vi "Import-Export_Service.vi"() -> ()   [LabVIEW 2014]
uses:
  _subVIs/_typedefs/impExp_Data.ctl
  <vilib>/NI Veristand/Templates/Workspace Tool Support/Workspace Tool Message Bus.ctl
  <vilib>/NI Veristand/Templates/Workspace Tool Support/Workspace Tool Message (String).ctl
  <vilib>/NI Veristand/Templates/Workspace Tool Support/Workspace Tool Response (String).ctl
  <vilib>/NI Veristand/Templates/Workspace Tool Support/Workspace Tool Message (Byte Array).ctl
  <vilib>/NI Veristand/Templates/Workspace Tool Support/Workspace Tool Response (Byte Array).ctl
  _subVIs/_typedefs/impExp_Service-StateData.ctl
  <vilib>/NI Veristand/Execution/Project/Project Ref.ctl
  _subVIs/Progress Bar/_typedefs/PB_Manager Actions.ctl
  <vilib>/NI/AMC/Create Single Message.vi
  <vilib>/NI/AMC/Update Message Routing Info.vi
  <vilib>/NI/AMC/Read Termination Message.vi
  <vilib>/NI/AMC/Send Message.vi
  <vilib>/NI/AMC/Globals.vi
  <vilib>/NI/AMC/AMC.lvlib
  NationalInstruments.VeriStand.ClientAPI
  <vilib>/NI Veristand/Execution/Project/NI_VS Project ExecutionAPI.lvlib
  <vilib>/NI VeriStand/Execution/Workspace/NI_VS Workspace ExecutionAPI.lvlib
  <vilib>/NI Veristand/Execution/Project/NI VeriStand - Send Workspace Tool Message (String).vi
  _subVIs/Progress Bar/Progress Bar.lvlib
  <vilib>/NI VeriStand/Templates/Workspace Tool Support/NI VeriStand - Workspace Tool Support.lvlib
panel:
  out "NIVS.Project File Path":path
  out "Workspace Events":i32
  in  "New Project/Screen Prefix":string="Proj1_MOD"
  out "Last update":string
  in  "Project/Screen to Import":path
  in  "Destination Folder":path
  in  "Import":bool
  in  "Export":bool
  out "SystemStateChange Events":i32
  in  "Data":T1
  in  "exit":bool
  # "Debug information"
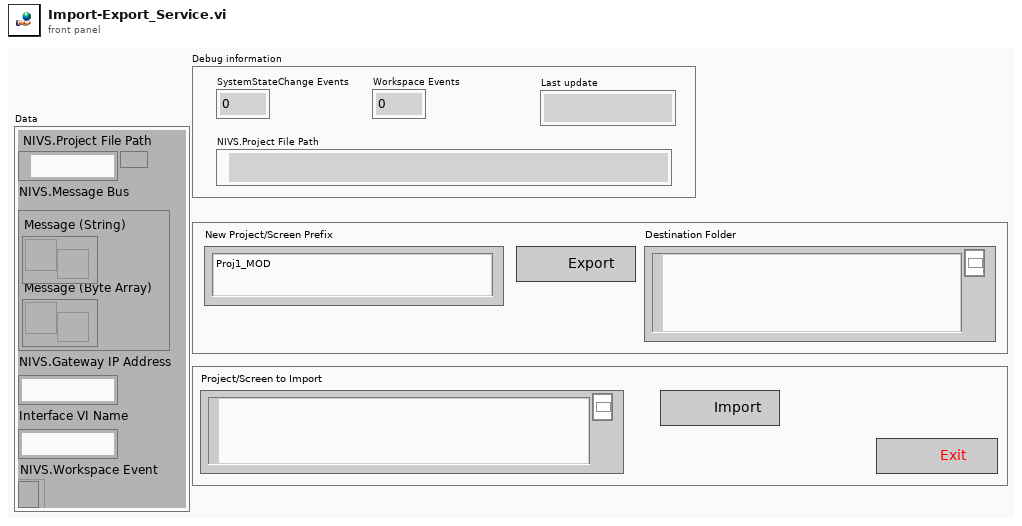
[diagram p1: front panel]
types:
  T1 = typedef "impExp_Data.ctl" = cluster{"NIVS.Project File Path":path, "NIVS.Message Bus":T2, "NIVS.Gateway IP Address":string, "Interface VI Name":string, "NIVS.Workspace Event":refnum<event-registration>}
  T2 = typedef "NI VeriStand - Workspace Tool Support.lvlib/Workspace Tool Message Bus.ctl" = cluster{"Message (String)":refnum<user-event>, "Message (Byte Array)":refnum<user-event>}
  T3 = typedef "impExp_Service-StateData.ctl" = cluster{"Source Project Path":path, "Destination Folder":path, "Name Prefix":string, "Project Ref":T4, "Shutdown":refnum<user-event>, "Interface VI Name":string}
  T4 = typedef "NI_VS Project ExecutionAPI.lvlib/Project Ref.ctl" = refnum<k24>
  T5 = typedef "NI_VS Workspace ExecutionAPI.lvlib/WorkspaceAPI.ctl" = refnum<k24>
  T6 = typedef "NI_VS Workspace ExecutionAPI.lvlib/SystemStateEventRef.ctl" = cluster{"CustDatRef":refnum<user-event>, "EvtRef":refnum<k27>}
  T7 = typedef "NI_VS Workspace ExecutionAPI.lvlib/SystemStateRegEventRef.ctl" = refnum<event-registration>
  T8 = typedef "AMC.lvlib/Message Queue.ctl" = refnum<queue>
  T9 = cluster{"Event Registration Refnum":refnum<event-registration>, "SystemChangeEventRef":T7, "Event Registration Refnum":refnum<event-registration>, "NIVS.Workspace Event":refnum<event-registration>}
  T10 = typedef "PB_Manager Actions.ctl" = enum16{"Init", "Update Bar", "Close"}
  T11 = typedef "AMC.lvlib/Message.ctl" = cluster{"name":string, "value":string, "attributes":T12, "receiver host":string, "receiver process":string, "source host":string, "source process":string, "priority message":bool, "acknowledge message":bool}
  T12 = typedef "Tools_KeyedArray.lvlib/KeyedArray.ctl" = cluster{"keys":string[], "values":string[]}
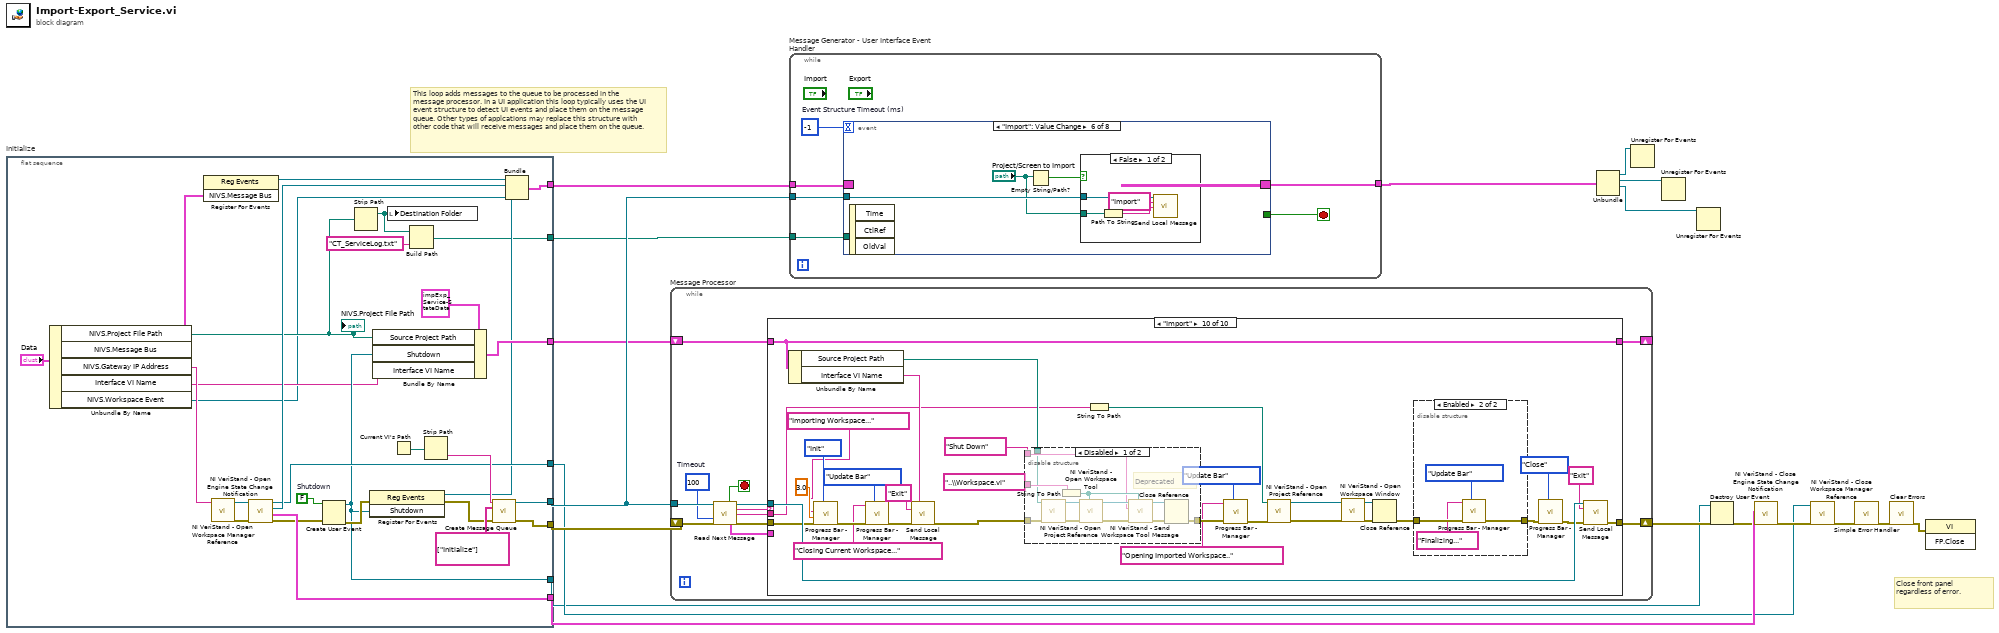
[diagram p0: block diagram]
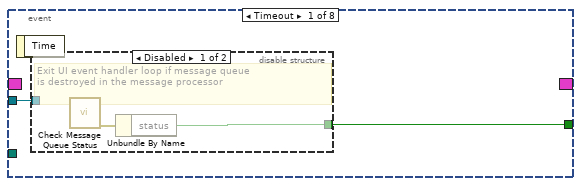
[diagram p2: hidden frame]
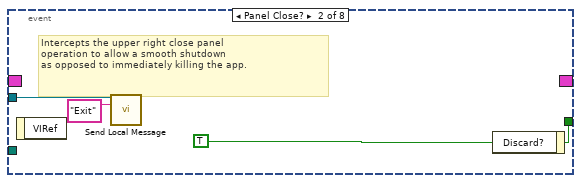
[diagram p4: hidden frame]
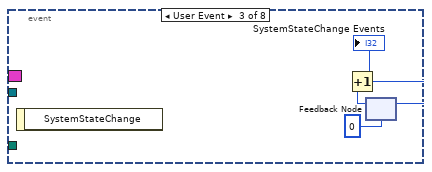
[diagram p5: hidden frame]
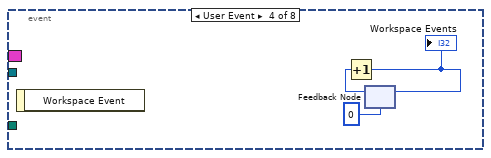
[diagram p6: hidden frame]
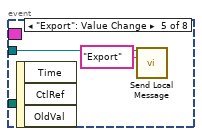
[diagram p7: hidden frame]
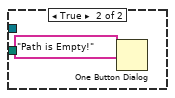
[diagram p8: hidden frame]
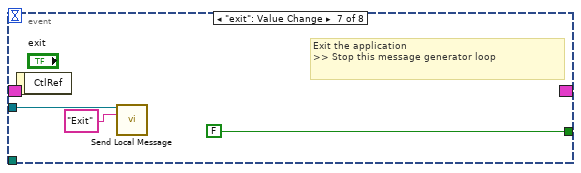
[diagram p9: hidden frame]
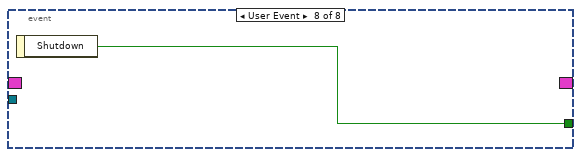
[diagram p10: hidden frame]
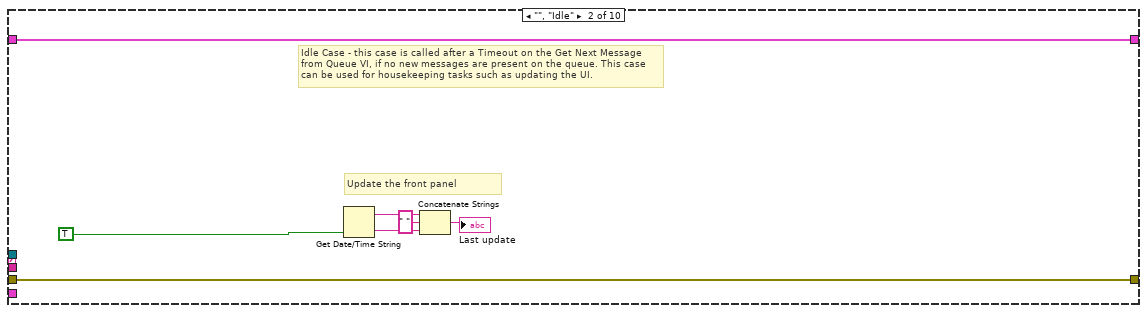
[diagram p12: hidden frame]
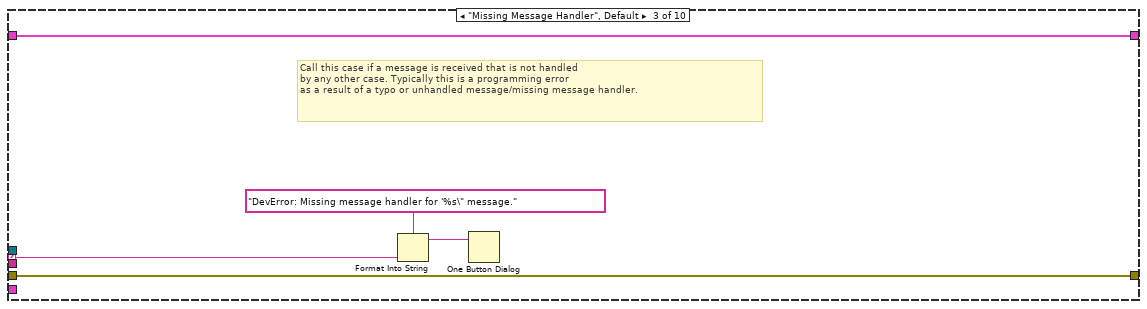
[diagram p13: hidden frame]
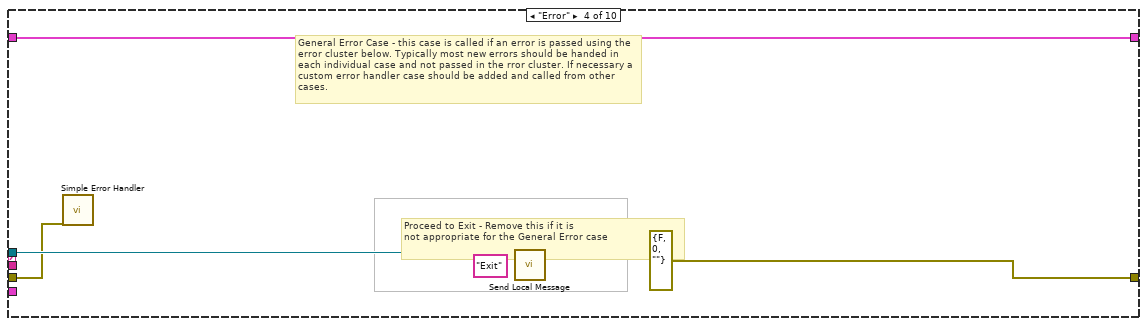
[diagram p14: hidden frame]
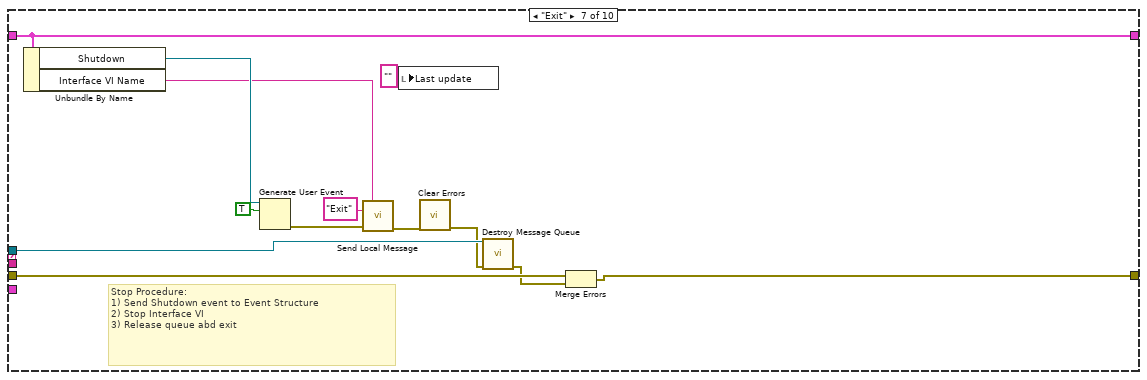
[diagram p17: hidden frame]
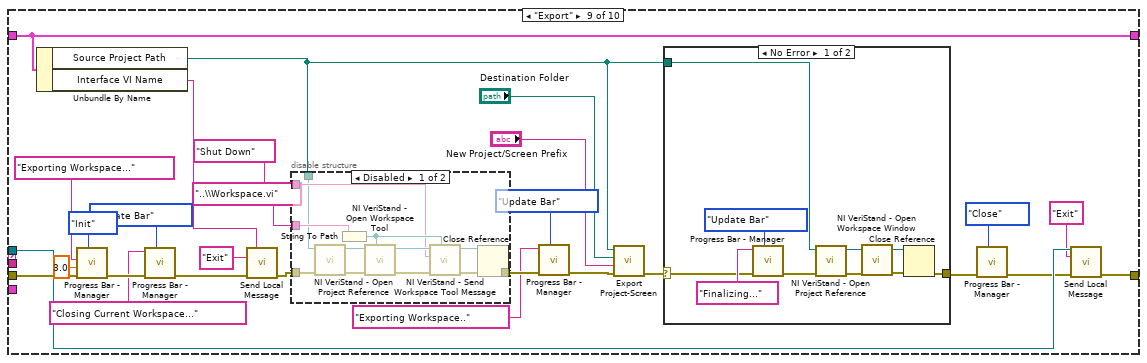
[diagram p19: hidden frame]
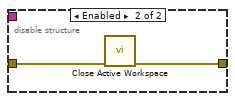
[diagram p20: hidden frame]
diagram:
  # "Close front panel\nregardless of error."
  # "This loop adds messages to the queue to be processed in the message processor. In a UI application this loop typically uses the UI event structure to detect UI events and place them on the message queue. Other types of applcations may replace this structure with other code that will receive messages and place them on the queue."
  n1 = flat-sequence "Initialize" {
    tunnel: [w45] -> w18
    tunnel: [w44] -> w17
    tunnel: [w40] -> w16
    tunnel: [w34] -> w14
    tunnel: [w32] -> w11
    tunnel: [w31] -> w13
    tunnel: [w24] -> w3
    tunnel: [w19] -> w1
    frame #0 {
      w29 = FALSE  # Shutdown
      n2 = Unbundle By Name("Data") -> ("NIVS.Project File Path"=w27:path, "NIVS.Message Bus"=w41:T2, "NIVS.Gateway IP Address"=w35:string, "Interface VI Name"=w23:string, "NIVS.Workspace Event"=w22:refnum<event-registration>)
      "NIVS.Project File Path" <- w27
      n3 = register-events(w41) -> (reference out=w38:refnum<event-registration>)  [unwired: 2 in, 1 out]
      n4 = call <vilib>:"NI VeriStand - Open Workspace Manager Reference.vi"("Gateway IP Address (\"\": localhost)"=w35) -> ("error out"=w37:errorcluster, "WorkspaceManager"=w36:T5)  [unwired: 9 in]
      n5 = call <vilib>:"NI VeriStand - Open Engine State Change Notification.vi"("error in (no error)"=w37, "WorkspaceManager in"=w36) -> ("error out"=w30:errorcluster, "SystemStateRefs"=w31:T6, "SystemChangeEventRef"=w33:T7, "WorkspaceManager out"=w32:T5)  [unwired: 6 in]
      n6 = Create User Event(user event datatype=w29, error in=w30) -> (user event=w24:refnum<user-event>, error out=w26:errorcluster)
      n7 = Strip Path(path=w27) -> (stripped path=w21:path)  [unwired: 1 out]
      n8 = register-events(error in=w26, w24) -> (reference out=w28:refnum<event-registration>, error out=w25:errorcluster)  [unwired: 1 in]
      n9 = Bundle By Name(cluster=T3 {"Source Project Path"=path "", "Destination Folder"=path "", "Name Prefix"="", "Project Ref"=refnum, "Shutdown"=refnum, "Interface VI Name"=""}, "Source Project Path"=w27, "Shutdown"=w24, "Interface VI Name"=w23) -> (w40:T3)
      n10 = local write "Destination Folder"(w21) -> ()
      n11 = Current VI's Path() -> (path=w43:path)
      n12 = Build Path(base path=w21, name or relative path="CT_ServiceLog.txt") -> (appended path=w19:path)
      n13 = Strip Path(path=w43) -> (name=w46:string)  [unwired: 1 out]
      n14 = call <vilib>:"Create Message Queue.vi"("message queue name"=w46, "initial message names"=string[] ["Initialize"], "error in"=w25) -> ("message queue out"=w45:T8, "error out"=w44:errorcluster)  [unwired: 11 in]
      n15 = Bundle("Event Registration Refnum"=w38, "SystemChangeEventRef"=w33, "Event Registration Refnum"=w28, "NIVS.Workspace Event"=w22) -> (w34:T9)  [unwired: 1 in]
    }
  }
  n16 = while "Message Processor" {
    shift-left: w17 -> [w53]
    shift-right: [w57] -> w4
    tunnel: w18 -> [w54]
    shift-left: w16 -> [w59]
    shift-right: [w58] -> _
    stop <- w56 stop-if-true
    w49 = 100  # Timeout
    n17 = call <vilib>:"Read Next Message.vi"("message queue in"=w54, "timeout (1 ms)"=w49, "error in"=w53) -> ("exit process?"=w56:bool, "message queue out"=w55:T8, "message name"=w51:string, "message value"=w50:string, "message"=w48:T11, "error out"=w52:errorcluster)  [unwired: 5 in, 2 out]
    n18 = case shown="\"Import\"" w51 {
      selector: w51 -> [_ _ w71 _ _ _ _ _ _ _]
      tunnel: [w61 w68 w73 w78 w80 w81 w92 w97 w125 w182] -> w58
      tunnel: w59 -> [w61 w68 w73 w78 w80 w81 w92 w97 w125 w182]
      tunnel: w55 -> [_ _ _ w76 _ _ w94 _ w103 w178]
      tunnel: w52 -> [w60 w67 w72 w74 w79 w82 w90 w96 w111 w166]
      tunnel: [w60 w67 w72 errorcluster {"status"=FALSE, "code"=0, "source"=""} ("error out") w79 w82 w88 w96 w101 w155] -> w57
      tunnel: w50 -> [_ _ _ _ _ _ _ _ _ w168]
      tunnel: w48 -> [_ _ _ _ _ _ _ _ _ _]
      frame "---------- Framework Operations ----------" {
        # "Dummy case to add a seperator in the Case Structure menu"
      }
      frame "", "Idle" {
        # "Update the front panel"
        # "Idle Case - this case is called after a Timeout on the Get Next Message from Queue VI, if no new messages are present on the queue. This case can be used for housekeeping tasks such as updating the UI."
        n19 = Get Date/Time String(want seconds? (F)=TRUE) -> (date string=w66:string, time string=w65:string)  [unwired: 2 out]
        n20 = Concatenate Strings(w66, " " ("string"), w65) -> (→"Last update":string)
      }
      frame "Missing Message Handler", Default {
        # "Call this case if a message is received that is not handled \nby any other case. Typically this is a programming error\nas a result of a typo or unhandled message/missing message handler."
        n21 = Format Into String(format string="DevError: Missing message handler for '%s\" message." ("message"), w71) -> (resulting string=w69:string)  [unwired: 2 in, 1 out]
        n22 = One Button Dialog(message=w69) -> ()  [unwired: 2 out]
      }
      frame "Error" {
        # "Proceed to Exit - Remove this if it is\nnot appropriate for the General Error case"
        # "General Error Case - this case is called if an error is passed using the error cluster below. Typically most new errors should be handed in each individual case and not passed in the rror cluster. If necessary a custom error handler case should be added and called from other cases."
        n23 = call <vilib>:"Simple Error Handler.vi"("error in (no error)"=w74) -> ()  [unwired: 1 in, 8 out]
        n24 = call <vilib>:"Send Local Message.vi"("message queue in"=w76, "message name"="Exit") -> ()  [unwired: 11 in, 3 out]
      }
      frame "---------- Generic Operations ----------" {
        # "Dummy case to add a seperator in the Case Structure menu"
      }
      frame "Initialize" {
      }
      frame "Exit" {
        # "Stop Procedure:\n1) Send Shutdown event to Event Structure\n2) Stop Interface VI\n3) Release queue abd exit"
        n25 = Unbundle By Name(w92) -> ("Shutdown"=w93:refnum<user-event>, "Interface VI Name"=w87:string)
        n26 = Generate User Event(user event=w93, event data cluster=TRUE ("event data")) -> (error out=w91:errorcluster)  [unwired: 2 in, 1 out]
        n27 = call <vilib>:"Send Local Message.vi"("receiver process (\"\" - local)"=w87, "message name"="Exit", "error in"=w91) -> ("error out"=w85:errorcluster)  [unwired: 10 in, 2 out]
        n28 = local write "Last update"("" ("Status")) -> ()
        n29 = call <vilib>:"Clear Errors.vi"("error in (no error)"=w85) -> ("error out"=w84:errorcluster)  [unwired: 5 in, 1 out]
        n30 = call <vilib>:"Destroy Message Queue.vi"("message queue in"=w94, "error in"=w84) -> ("error out"=w89:errorcluster)  [unwired: 11 in, 2 out]
        n31 = Merge Errors(w90, w89) -> (w88:errorcluster)
      }
      frame "---------- Application Operations ----------" {
        # "Dummy case to add a seperator in the Case Structure menu"
      }
      frame "Export" {
        n32 = Unbundle By Name(w125) -> ("Source Project Path"=w119:path, "Interface VI Name"=w116:string)
        n33 = call "Progress Bar - Manager.vi"("Action (Init)"=PB_Manager_Actions."Init", "error in (no error)"=w111, "Number of Steps"=3.0, "Window Title (\"\")"="Exporting Workspace..." ("Window Title (\"\")")) -> ("error out"=w115:errorcluster)  [unwired: 7 in]
        n34 = call "Progress Bar - Manager.vi"("Action (Init)"=PB_Manager_Actions."Update Bar", "error in (no error)"=w115, "Message"="Closing Current Workspace...") -> ("error out"=w110:errorcluster)  [unwired: 8 in]
        n35 = call <vilib>:"Send Local Message.vi"("receiver process (\"\" - local)"=w116, "message name"="Exit", "error in"=w110) -> ("error out"=w118:errorcluster)  [unwired: 10 in, 2 out]
        n36 = disable-structure shown="Disabled" {
          disable-tunnel: "..\\Workspace.vi" ("Custom Tool Path") -> [w134 _]
          disable-tunnel: "Shut Down" ("Command") -> [w133 _]
          disable-tunnel: w118 -> [w132 w139]
          disable-tunnel: [w127 w138] -> w109
          disable-tunnel: w119 -> [w131 _]
          frame Disabled {
            n37 = call <vilib>:"NI VeriStand - Open Project Reference.vi"("error in (no error)"=w132, "Project File Path"=w131) -> ("error out"=w129:errorcluster, "Project Ref"=w130:T4)  [unwired: 8 in]
            n38 = String To Path(string=w134) -> (path=w137:path)
            n39 = call <vilib>:"NI VeriStand - Open Workspace Tool.vi"("Workspace Tool Path"=w137, "error in (no error)"=w129, "Project Ref in"=w130) -> ("error out"=w136:errorcluster, "Project Ref out"=w135:T4)  [unwired: 7 in]
            n40 = call-poly <vilib>:"NI VeriStand - Send Workspace Tool Message.vi"("Workspace Tool Path"=w137, "error in (no error)"=w136, "Command"=w133, "Project Ref in"=w135) -> ("error out"=w128:errorcluster, "Project Ref out"=w126:T4)  [unwired: 5 in, 1 out]
            n41 = Close Reference(reference=w126, error in (no error)=w128) -> (error out=w127:errorcluster)
          }
          frame Enabled {
            n42 = call "Close Active Workspace.vi"("error in (no error)"=w139) -> ("error out"=w138:errorcluster)  [unwired: 10 in]
          }
        }
        n43 = call "Progress Bar - Manager.vi"("Action (Init)"=PB_Manager_Actions."Update Bar", "error in (no error)"=w109, "Message"="Exporting Workspace..") -> ("error out"=w108:errorcluster)  [unwired: 8 in]
        n44 = call "Export Project-Screen.vi"("error in (no error)"=w108, "File Prefix"="New Project/Screen Prefix", "Destination Folder"="Destination Folder", "File Path - Source"=w119) -> ("error out"=w120:errorcluster)  [unwired: 7 in]
        n45 = case shown="No Error" w120 {
          selector: w120 -> [w142 w150]
          tunnel: [w140 w150] -> w104
          tunnel: w119 -> [w147 _]
          frame No Error {
            n46 = call "Progress Bar - Manager.vi"("Action (Init)"=PB_Manager_Actions."Update Bar", "error in (no error)"=w142, "Message"="Finalizing...") -> ("error out"=w141:errorcluster)  [unwired: 8 in]
            n47 = call <vilib>:"NI VeriStand - Open Project Reference.vi"("error in (no error)"=w141, "Project File Path"=w147) -> ("error out"=w149:errorcluster, "Project Ref"=w146:T4)  [unwired: 8 in]
            n48 = call <vilib>:"NI VeriStand - Open Workspace Window.vi"("error in (no error)"=w149, "Project Ref in"=w146) -> ("error out"=w148:errorcluster, "Project Ref out"=w145:T4)  [unwired: 8 in]
            n49 = Close Reference(reference=w145, error in (no error)=w148) -> (error out=w140:errorcluster)
          }
          frame Error {
          }
        }
        n50 = call "Progress Bar - Manager.vi"("Action (Init)"=PB_Manager_Actions."Close", "error in (no error)"=w104) -> ("error out"=w102:errorcluster)  [unwired: 9 in]
        n51 = call <vilib>:"Send Local Message.vi"("message queue in"=w103, "message name"="Exit", "error in"=w102) -> ("error out"=w101:errorcluster)  [unwired: 10 in, 2 out]
      }
      frame "Import" {
        n52 = Unbundle By Name(w182) -> ("Source Project Path"=w179:path, "Interface VI Name"=w175:string)
        n53 = call "Progress Bar - Manager.vi"("Action (Init)"=PB_Manager_Actions."Init", "error in (no error)"=w166, "Number of Steps"=3.0, "Window Title (\"\")"="Importing Workspace..." ("Window Title (\"\")")) -> ("error out"=w165:errorcluster)  [unwired: 7 in]
        n54 = call "Progress Bar - Manager.vi"("Action (Init)"=PB_Manager_Actions."Update Bar", "error in (no error)"=w165, "Message"="Closing Current Workspace...") -> ("error out"=w164:errorcluster)  [unwired: 8 in]
        n55 = call <vilib>:"Send Local Message.vi"("receiver process (\"\" - local)"=w175, "message name"="Exit", "error in"=w164) -> ("error out"=w177:errorcluster)  [unwired: 10 in, 2 out]
        n56 = disable-structure shown="Disabled" {
          disable-tunnel: "..\\Workspace.vi" ("Custom Tool Path") -> [w199 _]
          disable-tunnel: "Shut Down" ("Command") -> [w198 _]
          disable-tunnel: w177 -> [w197 w204]
          disable-tunnel: [w192 w203] -> w160
          disable-tunnel: w179 -> [w196 _]
          frame Disabled {
            # "Deprecated"
            n57 = call <vilib>:"NI VeriStand - Open Project Reference.vi"("error in (no error)"=w197, "Project File Path"=w196) -> ("error out"=w194:errorcluster, "Project Ref"=w195:T4)  [unwired: 8 in]
            n58 = String To Path(string=w199) -> (path=w202:path)
            n59 = call <vilib>:"NI VeriStand - Open Workspace Tool.vi"("Workspace Tool Path"=w202, "error in (no error)"=w194, "Project Ref in"=w195) -> ("error out"=w201:errorcluster, "Project Ref out"=w200:T4)  [unwired: 7 in]
            n60 = call-poly <vilib>:"NI VeriStand - Send Workspace Tool Message.vi"("Workspace Tool Path"=w202, "error in (no error)"=w201, "Command"=w198, "Project Ref in"=w200) -> ("error out"=w193:errorcluster, "Project Ref out"=w191:T4)  [unwired: 5 in, 1 out]
            n61 = Close Reference(reference=w191, error in (no error)=w193) -> (error out=w192:errorcluster)
          }
          frame Enabled {
            n62 = call "Close Active Workspace.vi"("error in (no error)"=w204) -> ("error out"=w203:errorcluster)  [unwired: 10 in]
          }
        }
        n63 = String To Path(string=w168) -> (path=w167:path)
        n64 = call "Progress Bar - Manager.vi"("Action (Init)"=PB_Manager_Actions."Update Bar", "error in (no error)"=w160, "Message"="Opening Imported Workspace..") -> ("error out"=w158:errorcluster)  [unwired: 8 in]
        n65 = call <vilib>:"NI VeriStand - Open Project Reference.vi"("error in (no error)"=w158, "Project File Path"=w167) -> ("error out"=w174:errorcluster, "Project Ref"=w172:T4)  [unwired: 8 in]
        n66 = call <vilib>:"NI VeriStand - Open Workspace Window.vi"("error in (no error)"=w174, "Project Ref in"=w172) -> ("error out"=w173:errorcluster, "Project Ref out"=w171:T4)  [unwired: 8 in]
        n67 = Close Reference(reference=w171, error in (no error)=w173) -> (error out=w169:errorcluster)
        n68 = disable-structure shown="Enabled" {
          disable-tunnel: [w184 w188] -> w153
          disable-tunnel: w169 -> [w183 w189]
          frame Disabled {
            n69 = flat-sequence {
              tunnel: [w185] -> w184
              tunnel: w183 -> [w185]
              frame #0 {
                n70 = One Button Dialog(message="Import Complete!") -> ()  [unwired: 1 in, 1 out]
              }
            }
          }
          frame Enabled {
            n71 = call "Progress Bar - Manager.vi"("Action (Init)"=PB_Manager_Actions."Update Bar", "error in (no error)"=w189, "Message"="Finalizing...") -> ("error out"=w188:errorcluster)  [unwired: 8 in]
          }
        }
        n72 = call "Progress Bar - Manager.vi"("Action (Init)"=PB_Manager_Actions."Close", "error in (no error)"=w153) -> ("error out"=w152:errorcluster)  [unwired: 9 in]
        n73 = call <vilib>:"Send Local Message.vi"("message queue in"=w178, "message name"="Exit", "error in"=w152) -> ("error out"=w155:errorcluster)  [unwired: 10 in, 2 out]
      }
    }
  }
  n74 = while "Message Generator - User Interface Event Handler" {
    tunnel: w18 -> [w208]
    tunnel: [w207] -> w15
    tunnel: w14 -> [w206]
    tunnel: w1 -> [w205]
    stop <- w209 stop-if-true
    w210 = -1  # Event Structure Timeout (ms)
    n75 = event shown="[5] \"Import\": Value Change" {
      selector: w206 -> [_ _ _ _ _ _ _ _]
      dyn-events: [_ _ _ _ _ _ _ _] -> w207
      timeout: w210 -> [_ _ _ _ _ _ _ _]
      tunnel: [w211 w218 _ _ _ _ FALSE ("Discard?") w238] -> w209
      tunnel: w208 -> [w212 w216 _ _ w226 w229 w235 _]
      tunnel: w205 -> [_ _ _ _ _ _ _ _]
      event Timeout {
        n76 = event-data() -> ()  [unwired: 2 out]
        n77 = disable-structure shown="Disabled" {
          disable-tunnel: w212 -> [w214 _]
          disable-tunnel: [w213 _] -> w211
          frame Disabled {
            # "Exit UI event handler loop if message queue\nis destroyed in the message processor"
            n78 = call <vilib>:"Check Message Queue Status.vi"("message queue in"=w214) -> ("error out"=w215:errorcluster)  [unwired: 10 in, 4 out]
            n79 = Unbundle By Name(w215) -> ("status"=w213:bool)
          }
          frame Enabled {
          }
        }
      }
      event Panel Close? {
        w218 = TRUE ("Discard?")
        # "Intercepts the upper right close panel\noperation to allow a smooth shutdown\nas opposed to immediately killing the app."
        n80 = event-data() -> ()  [unwired: 2 out]
        n81 = call <vilib>:"Send Local Message.vi"("message queue in"=w216, "message name"="Exit") -> ()  [unwired: 11 in, 3 out]
        n82 = event-data("Discard?"=w218) -> ()  [unwired: 1 in, 1 out]
      }
      event User Event {
        n83 = event-data() -> ()  [unwired: 2 out]
        n84 = feedback #1(0) -> (w220:i32)
        n85 = Increment(x=w220) -> (x+1=w221:i32)
        "SystemStateChange Events" <- w221
        n86 = feedback-in #1(w221) -> ()
      }
      event User Event {
        n87 = event-data() -> ()  [unwired: 2 out]
        n88 = feedback #2(0) -> (w223:i32)
        n89 = Increment(x=w223) -> (x+1=w224:i32)
        "Workspace Events" <- w224
        n90 = feedback-in #2(w224) -> ()
      }
      event "Export": Value Change {
        n91 = event-data() -> ()  [unwired: 4 out]
        n92 = call <vilib>:"Send Local Message.vi"("message queue in"=w226, "message name"="Export") -> ()  [unwired: 11 in, 3 out]
      }
      event "Import": Value Change {
        n93 = event-data() -> ()  [unwired: 4 out]
        n94 = Empty String/Path?(string/path="Project/Screen to Import") -> (empty?=w228:bool)
        n95 = case shown="False" w228 {
          tunnel: w229 -> [w233 _]
          tunnel: "Project/Screen to Import" -> [w231 _]
          frame False {
            n96 = Path To String(path=w231) -> (string=w230:string)
            n97 = call <vilib>:"Send Local Message.vi"("message queue in"=w233, "message name"="Import", "message value"=w230) -> ()  [unwired: 10 in, 3 out]
          }
          frame True {
            n98 = One Button Dialog(message="Path is Empty!") -> ()  [unwired: 1 in, 1 out]
          }
        }
      }
      event "exit": Value Change {
        # "Exit the application\n>> Stop this message generator loop"
        n99 = event-data() -> ()  [unwired: 2 out]
        n100 = call <vilib>:"Send Local Message.vi"("message queue in"=w235, "message name"="Exit") -> ()  [unwired: 11 in, 3 out]
      }
      event User Event {
        n101 = event-data() -> ("Shutdown"=w238:bool)  [unwired: 1 out]
      }
    }
  }
  n102 = Unbundle(w15) -> ("Event Registration Refnum"=w10:refnum<event-registration>, "SystemChangeEventRef"=w9:T7, "Event Registration Refnum"=w5:refnum<event-registration>)  [unwired: 1 out]
  n103 = Unregister For Events(event registration refnum=w10) -> ()  [unwired: 1 in, 1 out]
  n104 = Unregister For Events(event registration refnum=w9) -> ()  [unwired: 1 in, 1 out]
  n105 = Unregister For Events(event registration refnum=w5) -> ()  [unwired: 1 in, 1 out]
  n106 = Destroy User Event(user event=w3, error in=w4) -> (error out=w2:errorcluster)
  n107 = call <vilib>:"NI VeriStand - Close Engine State Change Notification.vi"("error in (no error)"=w2, "SystemStateRefs"=w13) -> ("error out"=w12:errorcluster)  [unwired: 9 in]
  n108 = call <vilib>:"NI VeriStand - Close Workspace Manager Reference.vi"("error in (no error)"=w12, "WorkspaceManager"=w11) -> ("error out"=w6:errorcluster)  [unwired: 9 in]
  n109 = call <vilib>:"Simple Error Handler.vi"("error in (no error)"=w6) -> ("error out"=w8:errorcluster)  [unwired: 4 in, 4 out]
  n110 = call <vilib>:"Clear Errors.vi"("error in (no error)"=w8) -> ("error out"=w7:errorcluster)  [unwired: 5 in, 1 out]
  n111 = invoke class="VI" method="FP.Close"(error in=w7) -> ()  [unwired: 2 in, 3 out]
